vi "CalcTrueVoltageHaskell.vi"(0 "Pressure SP":dbl) -> (4 "Voltage":dbl)   [LabVIEW 2019, in "Stand.lvclass"]
uses:
  Stand.lvclass
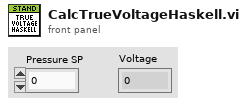
[diagram p1: front panel]
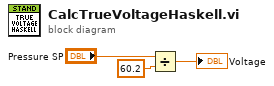
[diagram p0: block diagram]
diagram:
  n1 = Divide(x="Pressure SP", y=60.2 ("x")) -> (x/y=→"Voltage":dbl)
